vi "PCO_CleanupLensControl.vi"(8 "error in (no error)":errorcluster {"code" format="%x"}) -> (0 "error out":errorcluster {"code" format="%x"}, 3 "ErrorMessage":i32 format="%x")   [LabVIEW 2020, in "SDK.lvlib" / "LensControl.lvlib"]
doc: "<b>Description:</b>\nCleans up all internal lens control objects, which were created. It closes and deletes all lens control objects.\nThis is an internally used helper function, which is also exported.\n\n<b>Supported camera type:</b>\npco.edge CLHS, pco.dimax cs\n\n<b>Descriptor dependency:</b>\nNone"
uses:
  LensControl.lvlib
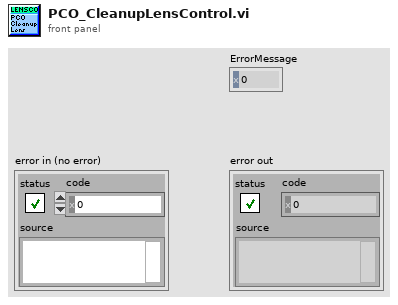
[diagram p1: front panel]
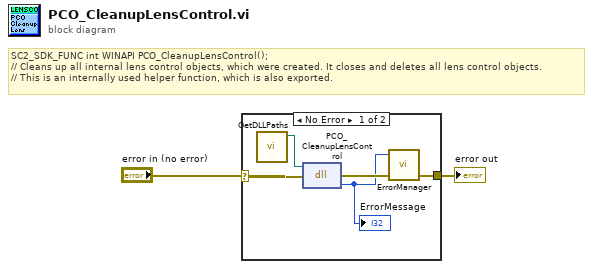
[diagram p0: block diagram]
diagram:
  # "SC2_SDK_FUNC int WINAPI PCO_CleanupLensControl();\n// Cleans up all internal lens control objects, which were created. It closes and deletes all lens control objects.\n// This is an internally used helper function, which is also exported."
  n1 = case shown="No Error" "error in (no error)" {
    selector: "error in (no error)" -> [w7 w8]
    tunnel: [w6 w8] -> w2
    frame No Error {
      n2 = call "GetDLLPaths.vi"() -> ("SC2_Cam_Path"=w3:path)  [unwired: 9 in, 2 out]
      n3 = dll-call lib="?" fn="PCO_CleanupLensControl"(path in=w3, error in=w7) -> (error out=w5:errorcluster, "return type"=w4:i32)  [unwired: 1 in, 1 out]
      "ErrorMessage" <- w4
      n4 = call "ErrorManager.vi"("error in (no error)"=w5, "error code"=w4) -> ("error out"=w6:errorcluster)  [unwired: 3 in]
    }
    frame Error {
    }
  }
  "error out" <- w2
